vi "校准数据选择表.vi"(10 "测量模式":T1(ring), 11 "table":string="CODMn") -> (2 "布尔":bool=TRUE, 3 "输出":T2)   [LabVIEW 2016, in "斯坦道总磷总氮.lvlib"]
uses:
  <vilib>/Utility/miscctls.llb/LVPointTypeDef.ctl
  <vilib>/Utility/miscctls.llb/LVRowAndColumnUnsignedTypeDef.ctl
panel:
  in  "确定":bool
  in  "返回":bool
  in  "多列列表框":i32(listbox)
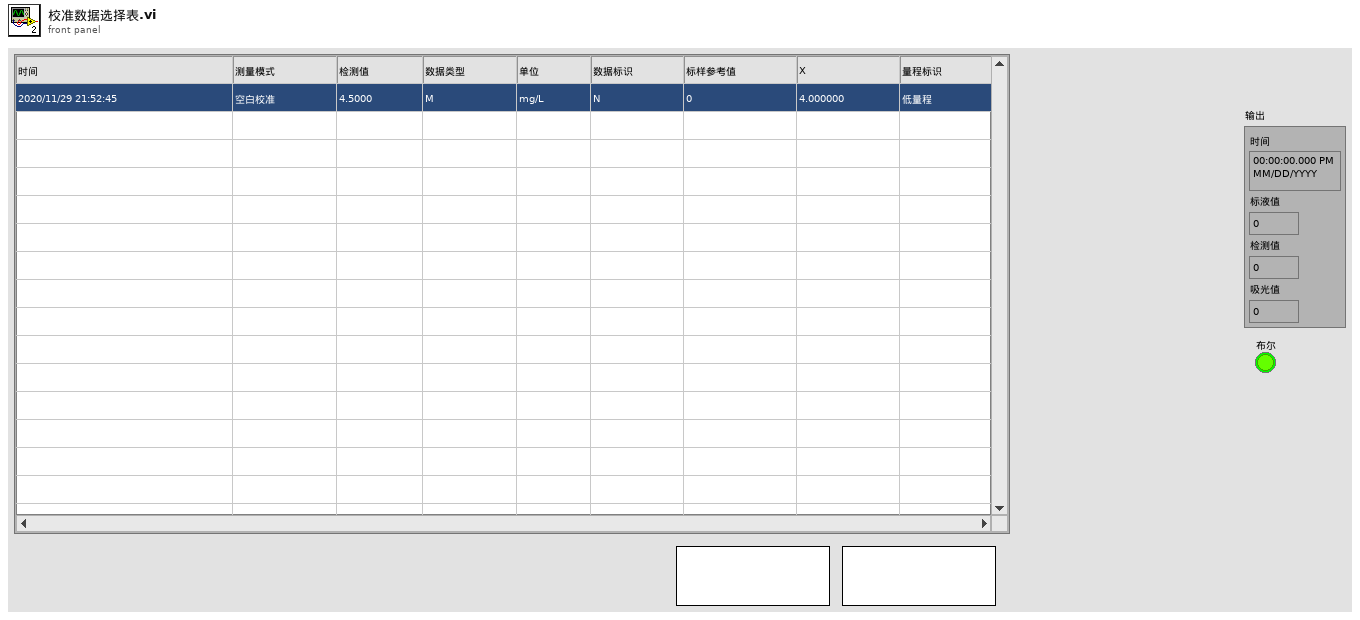
[diagram p1: front panel]
types:
  T1 = enum16{"跨度核查", "水样测量", "零点核查", "标样核查", "加标回收", "快捷测试", "空白校准", "标样校准"}
  T2 = cluster{"时间":timestamp, "标液值":dbl, "检测值":dbl, "吸光值":dbl}
  T3 = typedef "LVRowAndColumnUnsignedTypeDef.ctl" = cluster{"Row":u32, "Column":u32}
  T4 = typedef "LVPointTypeDef.ctl" = cluster{"Horizontal":i16, "Vertical":i16}
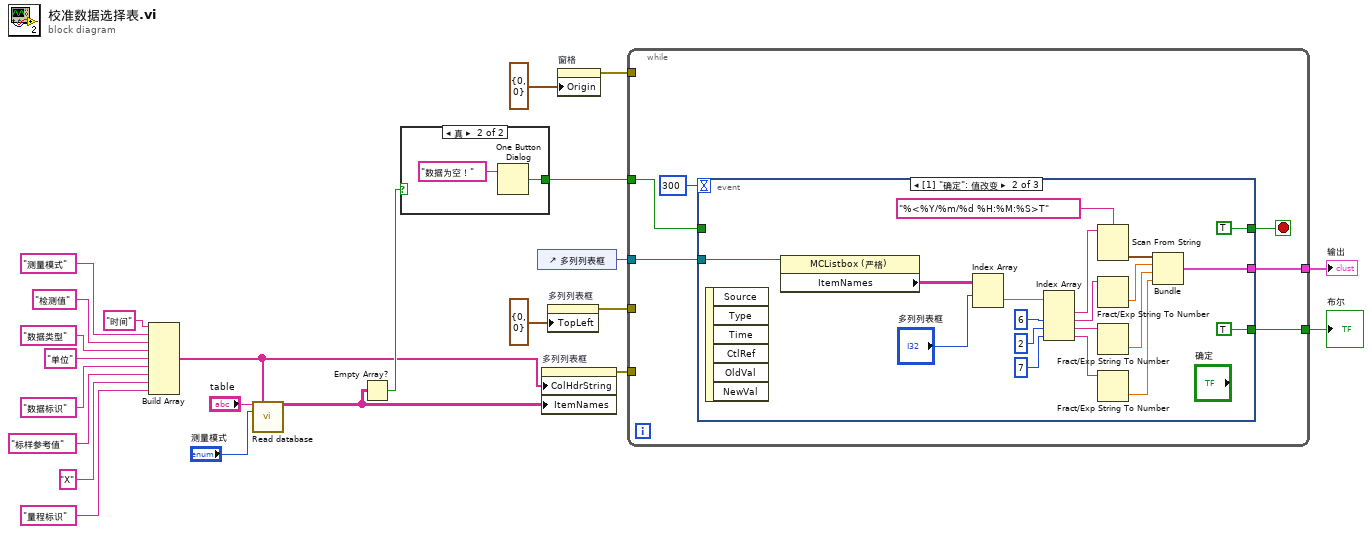
[diagram p0: block diagram]
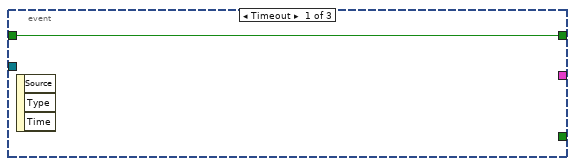
[diagram p3: hidden frame]
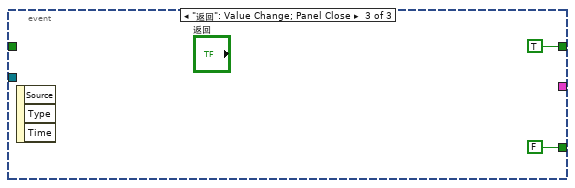
[diagram p4: hidden frame]
diagram:
  n1 = Build Array("时间", "测量模式", "检测值", "数据类型", "单位", "数据标识", "标样参考值", "X", "量程标识") -> (w9:string[])
  n2 = call "Read database.vi"("table"="table", "显示项"=w9, "测量模式"="测量模式") -> ("表格"=w19:string[][])  [unwired: 9 in, 3 out]
  n3 = Empty Array?(array=w19) -> (empty?=w18:bool)
  n4 = case shown="真" w18 {
    tunnel: [_ w24] -> w17
    frame False {
    }
    frame True {
      n5 = One Button Dialog(message="数据为空！" ("消息")) -> (true=w24:bool)  [unwired: 1 in]
    }
  }
  n6 = control-ref of="多列列表框"() -> (w3:refnum<vi>)
  n7 = property on="多列列表框" class="MCListbox (严格)"("ColHdrString"=w9, "ItemNames"=w19) -> (error out=w20:errorcluster)  [unwired: 2 in, 1 out]
  n8 = property on="多列列表框" class="MCListbox (严格)"("TopLeft"=T3 {"Row"=0, "Column"=0} ("左上可见单元格")) -> (error out=w1:errorcluster)  [unwired: 2 in, 1 out]
  n9 = property on="窗格" class="Pane"("Origin"=T4 {"Horizontal"=0, "Vertical"=0} ("原点")) -> (error out=w22:errorcluster)  [unwired: 2 in, 1 out]
  n10 = while {
    tunnel: w3 -> [w30]
    tunnel: w22 -> [_]
    tunnel: [w29] -> w21
    tunnel: w20 -> [_]
    tunnel: w17 -> [w28]
    tunnel: [w26] -> w7
    tunnel: w1 -> [_]
    stop <- w31 stop-if-true
    n11 = event shown="[1] \"确定\": 值改变" {
      selector: _ -> [_ _ _]
      dyn-events: _ -> [_ _ _]
      timeout: 300 -> [_ _ _]
      tunnel: [w32 TRUE TRUE] -> w31
      tunnel: w30 -> [_ w49 _]
      tunnel: [_ TRUE FALSE] -> w29
      tunnel: w28 -> [w32 _ _]
      tunnel: [_ w36 _] -> w26
      event Timeout {
        n12 = event-data() -> ()  [unwired: 1 in, 3 out]
      }
      event "确定": Value Change {
        n13 = event-data() -> ()  [unwired: 1 in, 6 out]
        n14 = property class="MCListbox (严格)"(reference=w49) -> ("ItemNames"=w50:string[][])  [unwired: 1 in, 2 out]
        n15 = Index Array(array=w50, index (row)="多列列表框") -> (element=w46:string[])  [unwired: 1 in]
        n16 = Index Array(array=w46, index #2=6 ("索引"), index #3=2 ("索引"), index #4=7 ("索引")) -> (element #1=w34:string, element #2=w42:string, element #3=w41:string, element #4=w40:string)  [unwired: 1 in]
        n17 = Scan From String(format string="%<%Y/%m/%d %H:%M:%S>T" ("格式字符串"), input string=w34) -> (output 1=w33:timestamp)  [unwired: 3 in, 3 out]
        n18 = Fract/Exp String To Number(string=w42) -> (number=w39:dbl)  [unwired: 3 in, 1 out]
        n19 = Fract/Exp String To Number(string=w41) -> (number=w38:dbl)  [unwired: 3 in, 1 out]
        n20 = Fract/Exp String To Number(string=w40) -> (number=w37:dbl)  [unwired: 3 in, 1 out]
        n21 = Bundle(w33, w39, w38, w37) -> (w36:cluster{timestamp, dbl, dbl, dbl})  [unwired: 1 in]
      }
      event "返回": Value Change; Panel Close {
        n22 = event-data() -> ()  [unwired: 1 in, 3 out]
      }
    }
  }
  "布尔" <- w21
  "输出" <- w7
